vi "AC_Test.vi"(1 "INData":string[](array[string])) -> (15 "OutData":string[](array[string]), 16 "结果数组":bool[](array[boolean]), 17 "读取缓冲区":string)   [LabVIEW 2018]
uses:
  Subvi/Global.vi
  <vilib>/Instr/_visa.llb/VISA Configure Serial Port (Instr).vi
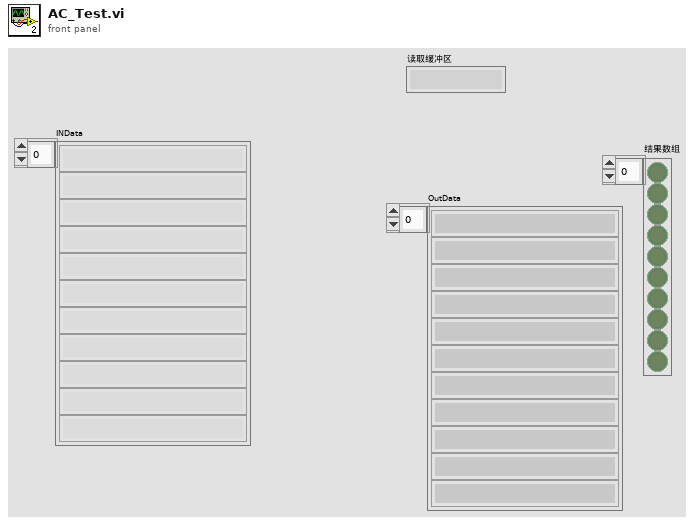
[diagram p1: front panel]
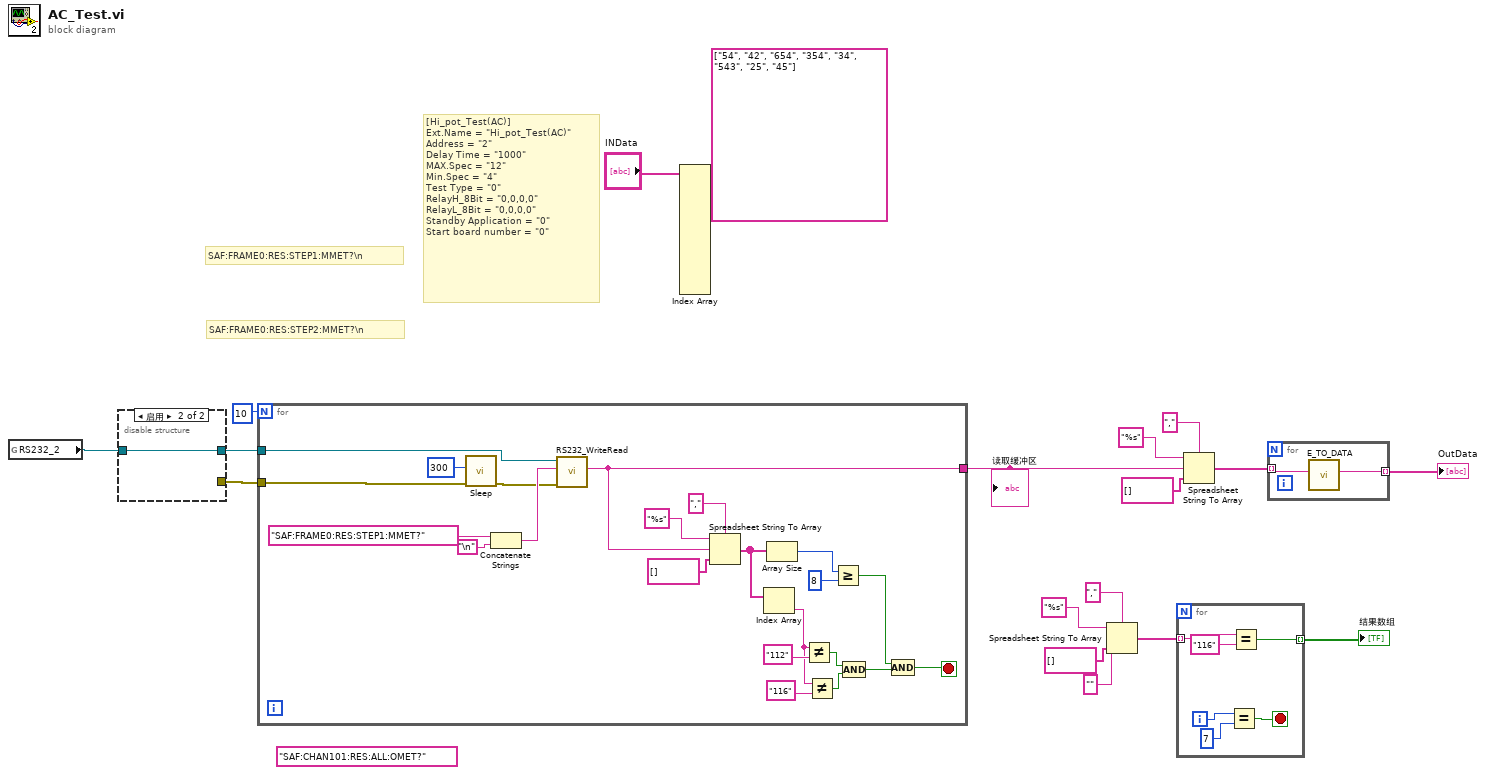
[diagram p0: block diagram]
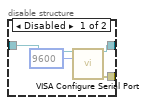
[diagram p2: hidden frame]
diagram:
  (unwired) "SAF:CHAN101:RES:ALL:OMET?" ("写入缓冲区")
  (unwired) string[] ["54", "42", "654", "354", "34", "543", "25", "45"]
  # "SAF:FRAME0:RES:STEP2:MMET?\\n"
  # "SAF:FRAME0:RES:STEP1:MMET?\\n"
  # "[Hi_pot_Test(AC)]\nExt.Name = \"Hi_pot_Test(AC)\"\nAddress = \"2\"\nDelay Time = \"1000\"\nMAX.Spec = \"12\"\nMin.Spec = \"4\"\nTest Type = \"0\"\nRelayH_8Bit = \"0,0,0,0\"\nRelayL_8Bit = \"0,0,0,0\"\nStandby Application = \"0\"\nStart board number = \"0\""
  n1 = global read "Global.vi" "RS232_2"() -> (w8:refnum<visa-resource-name>)
  n2 = disable-structure shown="启用" {
    disable-tunnel: w8 -> [w21 w22]
    disable-tunnel: [w20 w22] -> w7
    disable-tunnel: [w18 _] -> w6
    frame Disabled {
      n3 = call-poly "VISA Configure Serial Port"("VISA resource name"=w21, "baud rate (9600)"=u32 9600) -> ("VISA resource name out"=w20:refnum<visa-resource-name>, "error out"=w18:errorcluster)  [unwired: 12 in]
    }
    frame Enabled {
    }
  }
  n4 = for {
    N: 10 -> [_]
    tunnel: [w34] -> w2
    tunnel: w7 -> [w39]
    tunnel: w6 -> [w38]
    stop <- w23 stop-if-true
    n5 = call "Sleep.vi"("error in (no error)"=w38, "等待时间（毫秒）"=u32 300) -> ("error out"=w40:errorcluster)  [unwired: 9 in]
    n6 = Concatenate Strings("SAF:FRAME0:RES:STEP1:MMET?" ("写入缓冲区"), "\n") -> (w42:string)
    n7 = call "RS232_WriteRead.vi"("错误输入（无错误）"=w40, "写入缓冲区"=w42, "VISA资源名称"=w39) -> ("读取缓冲区"=w34:string)  [unwired: 6 in, 2 out]
    n8 = Spreadsheet String To Array(delimiter (Tab)="," ("分隔符(Tab)"), format string="%s" ("电子表格字符串"), spreadsheet string=w34, array type (2D Dbl)=string[] []) -> (array=w31:string[])
    n9 = Index Array(array=w31) -> (element=w28:string)  [unwired: 1 in]
    n10 = Array Size(array=w31) -> (size(s)=w33:i32)
    n11 = Not Equal?(x=w28, y="112") -> (x != y?=w27:bool)
    n12 = Not Equal?(x=w28, y="116") -> (x != y?=w26:bool)
    n13 = Greater Or Equal?(x=w33, y=8) -> (x >= y?=w24:bool)
    n14 = Compound Arithmetic op=AND ("复合运算")(w27, w26) -> (w25:bool)
    n15 = Compound Arithmetic op=AND ("复合运算")(w24, w25) -> (w23:bool)
  }
  "读取缓冲区" <- w2
  n16 = Index Array(array="INData") -> ()  [unwired: 14 in, 14 out]
  n17 = Spreadsheet String To Array(delimiter (Tab)="," ("分隔符(Tab)"), format string="%s" ("电子表格字符串"), spreadsheet string="" ("电子表格字符串"), array type (2D Dbl)=string[] []) -> (array=w13:string[])
  n18 = for {
    tunnel: w13 -> [w47] mode=indexing
    tunnel: [w45] -> w12 mode=indexing
    i -> [w49]
    stop <- w48 stop-if-true
    n19 = Equal?(x=w49, y=7) -> (x = y?=w48:bool)
    n20 = Equal?(x=w47, y="116") -> (x = y?=w45:bool)
  }
  "结果数组" <- w12
  n21 = Spreadsheet String To Array(delimiter (Tab)="," ("分隔符(Tab)"), format string="%s" ("电子表格字符串"), spreadsheet string=w2, array type (2D Dbl)=string[] []) -> (array=w5:string[])
  n22 = for {
    tunnel: w5 -> [w52] mode=indexing
    tunnel: [w51] -> w4 mode=indexing
    n23 = call "E_TO_DATA.vi"("INPUT"=w52) -> ("F-格式字符串"=w51:string)  [unwired: 9 in, 1 out]
  }
  "OutData" <- w4
